vi "weight adjustment.vi"(1 "Learning Rate":dbl=1.0, 2 "Error":dbl[](array[numeric]), 3 "Weight":dbl[][](array[numeric]), 4 "Input":dbl[](array[numeric])) -> (0 "Weight out":dbl[][](array[numeric]))   [LabVIEW 2009]
uses:
  <vilib>/Analysis/Matrix/Numeric/Conversions/Matrix To Array - RM.vi
  <vilib>/Analysis/Matrix/Numeric/Add/Add - RM,RM.vi
  <vilib>/Analysis/Matrix/Numeric/Conversions/Array To Matrix - RA2.vi
  <vilib>/Analysis/Matrix/Numeric/Multiply/Multiply - RM,R.vi
  <vilib>/Analysis/Matrix/Numeric/Multiply/Multiply - RM,RM.vi
  <vilib>/Analysis/Matrix/Numeric/Conversions/Array To Matrix - RA.vi
  <vilib>/Analysis/Matrix/NI_Matrix.lvlib
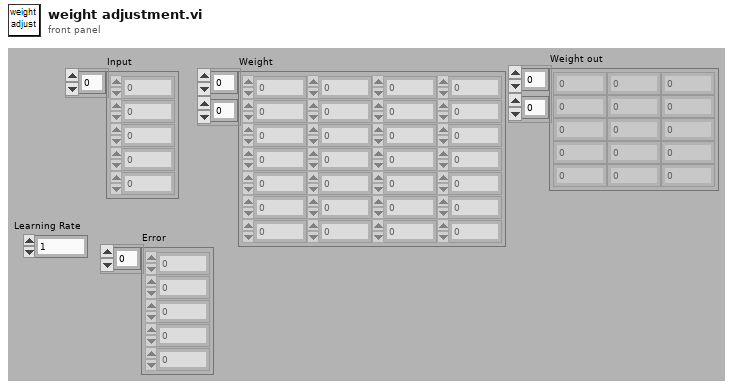
[diagram p1: front panel]
types:
  T1 = typedef "NI_Matrix.lvlib/RealMatrix.ctl" = dbl[][]
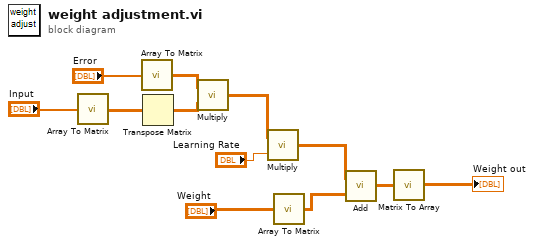
[diagram p0: block diagram]
diagram:
  n1 = call-poly <vilib>:"Array To Matrix.vi"("Real 1D Array"="Input") -> ("Real Matrix (Column Vector)"=w11:T1)
  n2 = call-poly <vilib>:"Array To Matrix.vi"("Real 1D Array"="Error") -> ("Real Matrix (Column Vector)"=w9:T1)
  n3 = Transpose Matrix(1:w11) -> (0:w8:T1)
  n4 = call-poly <vilib>:"Multiply.vi"("Real Matrix B"=w8, "Real Matrix A"=w9) -> ("A * B"=w6:T1)
  n5 = call-poly <vilib>:"Multiply.vi"("Real Scalar c"="Learning Rate", "Real Matrix A"=w6) -> ("A * c"=w4:T1)
  n6 = call-poly <vilib>:"Array To Matrix.vi"("Real 2D Array"="Weight") -> ("Real Matrix"=w5:T1)
  n7 = call-poly <vilib>:"Add.vi"("Real Matrix B"=w5, "Real Matrix A"=w4) -> ("A + B"=w3:T1)
  n8 = call-poly <vilib>:"Matrix To Array.vi"("Real Matrix"=w3) -> ("Real 2D Array"=→"Weight out":dbl[][])
